vi "rsidr_core_global.vi"() -> ()   [LabVIEW 2020, in "Rohde&Schwarz RTx Oscilloscopes.lvlib"] (continued)
2"=0.0, "Command"="DESK"}]}, {"Type"=2, "Name"="rsrtx_rngScaleLinLog", "Entries"=[{"Name"="Linear", "Value 1"=0.0, "Value 2"=0.0, "Command"="LIN"}, {"Name"="Logarithmic", "Value 1"=1.0, "Value 2"=0.0, "Command"="LOG"}]}, {"Type"=2, "Name"="rsrtx_rngHarmonicsFundamentalMIL", "Entries"=[{"Name"="F60", "Value 1"=0.0, "Value 2"=0.0, "Command"="F60"}, {"Name"="F400", "Value 1"=1.0, "Value 2"=0.0, "Command"="F400"}]}, {"Type"=2, "Name"="rsrtx_rngHarmonicsFundamentalRTC", "Entries"=[{"Name"="F400", "Value 1"=0.0, "Value 2"=0.0, "Command"="F400"}, {"Name"="NVF", "Value 1"=1.0, "Value 2"=0.0, "Command"="NVF"}, {"Name"="WVF", "Value 1"=2.0, "Value 2"=0.0, "Command"="WVF"}]}, {"Type"=0, "Name"="rsrtx_rngPowerAnalysisReportTemperature", "Entries"=[{"Name"="", "Value 1"=-273.0, "Value 2"=32767.0, "Command"=""}]}, {"Type"=0, "Name"="rsrtx_rngTransientResponseSignal", "Entries"=[{"Name"="", "Value 1"=-10.0, "Value 2"=10.0, "Command"=""}]}, {"Type"=2, "Name"="rsrtx_rngProbeInputImpedance", "Entries"=[{"Name"="Unknown termination", "Value 1"=0.0, "Value 2"=0.0, "Command"="UNKN"}, {"Name"="50 Ohm termination", "Value 1"=1.0, "Value 2"=0.0, "Command"="50OH"}, {"Name"="1 M Ohm termination", "Value 1"=2.0, "Value 2"=0.0, "Command"="1MOH"}]}, {"Type"=2, "Name"="RsRtx_rngClockedSource", "Entries"=[{"Name"="D0", "Value 1"=0.0, "Value 2"=0.0, "Command"="D0"}, {"Name"="D1", "Value 1"=1.0, "Value 2"=0.0, "Command"="D1"}, {"Name"="D2", "Value 1"=2.0, "Value 2"=0.0, "Command"="D2"}, {"Name"="D3", "Value 1"=3.0, "Value 2"=0.0, "Command"="D3"}, {"Name"="D4", "Value 1"=4.0, "Value 2"=0.0, "Command"="D4"}, {"Name"="D5", "Value 1"=5.0, "Value 2"=0.0, "Command"="D5"}, {"Name"="D6", "Value 1"=6.0, "Value 2"=0.0, "Command"="D6"}, {"Name"="D7", "Value 1"=7.0, "Value 2"=0.0, "Command"="D7"}, {"Name"="D8", "Value 1"=8.0, "Value 2"=0.0, "Command"="D8"}, {"Name"="D9", "Value 1"=9.0, "Value 2"=0.0, "Command"="D9"}, {"Name"="D10", "Value 1"=10.0, "Value 2"=0.0, "Command"="D10"}, {"Name"="D11", "Value 1"=11.0, "Value 2"=0.0, "Command"="D11"}, {"Name"="D12", "Value 1"=12.0, "Value 2"=0.0, "Command"="D12"}, {"Name"="D13", "Value 1"=13.0, "Value 2"=0.0, "Command"="D13"}, {"Name"="D14", "Value 1"=14.0, "Value 2"=0.0, "Command"="D14"}, {"Name"="D15", "Value 1"=15.0, "Value 2"=0.0, "Command"="D15"}]}, {"Type"=2, "Name"="RsRtx_rngParallelBitSource", "Entries"=[{"Name"="D0", "Value 1"=0.0, "Value 2"=0.0, "Command"="D0"}, {"Name"="D1", "Value 1"=1.0, "Value 2"=0.0, "Command"="D1"}, {"Name"="D2", "Value 1"=2.0, "Value 2"=0.0, "Command"="D2"}, {"Name"="D3", "Value 1"=3.0, "Value 2"=0.0, "Command"="D3"}, {"Name"="D4", "Value 1"=4.0, "Value 2"=0.0, "Command"="D4"}, {"Name"="D5", "Value 1"=5.0, "Value 2"=0.0, "Command"="D5"}, {"Name"="D6", "Value 1"=6.0, "Value 2"=0.0, "Command"="D6"}, {"Name"="D7", "Value 1"=7.0, "Value 2"=0.0, "Command"="D7"}, {"Name"="D8", "Value 1"=8.0, "Value 2"=0.0, "Command"="D8"}, {"Name"="D9", "Value 1"=9.0, "Value 2"=0.0, "Command"="D9"}, {"Name"="D10", "Value 1"=10.0, "Value 2"=0.0, "Command"="D10"}, {"Name"="D11", "Value 1"=11.0, "Value 2"=0.0, "Command"="D11"}, {"Name"="D12", "Value 1"=12.0, "Value 2"=0.0, "Command"="D12"}, {"Name"="D13", "Value 1"=13.0, "Value 2"=0.0, "Command"="D13"}, {"Name"="D14", "Value 1"=14.0, "Value 2"=0.0, "Command"="D14"}, {"Name"="D15", "Value 1"=15.0, "Value 2"=0.0, "Command"="D15"}]}, {"Type"=0, "Name"="RsRtx_rngPctInt", "Entries"=[{"Name"="", "Value 1"=0.0, "Value 2"=100.0, "Command"=""}]}, {"Type"=2, "Name"="RsRtx_rngDVMType", "Entries"=[{"Name"="DC", "Value 1"=0.0, "Value 2"=0.0, "Command"="DC"}, {"Name"="AC DC RMS", "Value 1"=1.0, "Value 2"=0.0, "Command"="ACDC"}, {"Name"="AC RMS", "Value 1"=2.0, "Value 2"=0.0, "Command"="ACRM"}, {"Name"="Maximum", "Value 1"=3.0, "Value 2"=0.0, "Command"="UPE"}, {"Name"="Minimum", "Value 1"=4.0, "Value 2"=0.0, "Command"="LPE"}, {"Name"="Peak-to-Peak", "Value 1"=5.0, "Value 2"=0.0, "Command"="PEAK"}, {"Name"="Crest Factor", "Value 1"=6.0, "Value 2"=0.0, "Command"="CRES"}, {"Name"="Off", "Value 1"=7.0, "Value 2"=0.0, "Command"="OFF"}]}, {"Type"=2, "Name"="RsRtx_rngDVMPosition", "Entries"=[{"Name"="Top Left Corner", "Value 1"=0.0, "Value 2"=0.0, "Command"="TLEF"}, {"Name"="Top Right Corner", "Value 1"=1.0, "Value 2"=0.0, "Command"="TRIG"}, {"Name"="Bottom Left Corner", "Value 1"=2.0, "Value 2"=0.0, "Command"="BLEF"}, {"Name"="Bottom Right Corner", "Value 1"=3.0, "Value 2"=0.0, "Command"="BRIG"}]}, {"Type"=2, "Name"="RsRtx_rngMagnitudeScale", "Entries"=[{"Name"="Linear", "Value 1"=0.0, "Value 2"=0.0, "Command"="LIN"}, {"Name"="dBM", "Value 1"=1.0, "Value 2"=0.0, "Command"="DBM"}, {"Name"="dBV", "Value 1"=2.0, "Value 2"=0.0, "Command"="DBV"}, {"Name"="dBuV", "Value 1"=3.0, "Value 2"=0.0, "Command"="DBUV"}]}, {"Type"=2, "Name"="RsRtx_rngSpectrumFrequencyWindowType", "Entries"=[{"Name"="Rectangular", "Value 1"=0.0, "Value 2"=0.0, "Command"="RECT"}, {"Name"="Hamming", "Value 1"=1.0, "Value 2"=0.0, "Command"="HAMM"}, {"Name"="Hanning", "Value 1"=2.0, "Value 2"=0.0, "Command"="HANN"}, {"Name"="Blackman Harris", "Value 1"=3.0, "Value 2"=0.0, "Command"="BLAC"}, {"Name"="Flat Top", "Value 1"=4.0, "Value 2"=0.0, "Command"="FLAT"}]}, {"Type"=0, "Name"="RsRtx_rngSpectrumSpectrogramScale", "Entries"=[{"Name"="", "Value 1"=1.0, "Value 2"=20.0, "Command"=""}]}, {"Type"=2, "Name"="RsRtx_rngSpectrumMarkerDisplay", "Entries"=[{"Name"="Off", "Value 1"=0.0, "Value 2"=0.0, "Command"="OFF"}, {"Name"="Index", "Value 1"=1.0, "Value 2"=0.0, "Command"="IND"}, {"Name"="Result", "Value 1"=2.0, "Value 2"=0.0, "Command"="RES"}]}, {"Type"=2, "Name"="RsRtx_rngSpectrumMarkerSource", "Entries"=[{"Name"="Spectrum", "Value 1"=0.0, "Value 2"=0.0, "Command"="SPEC"}, {"Name"="Min Hold", "Value 1"=1.0, "Value 2"=0.0, "Command"="MINH"}, {"Name"="Max Hold", "Value 1"=2.0, "Value 2"=0.0, "Command"="MAXH"}, {"Name"="Average", "Value 1"=3.0, "Value 2"=0.0, "Command"="AVER"}]}, {"Type"=2, "Name"="RsRtx_rngSpectrumMarkerSetupDetectionMode", "Entries"=[{"Name"="Level Only", "Value 1"=0.0, "Value 2"=0.0, "Command"="LONL"}, {"Name"="Advanced", "Value 1"=1.0, "Value 2"=0.0, "Command"="ADV"}]}, {"Type"=2, "Name"="RsRtx_rngSpectrumMarkerReferenceMode", "Entries"=[{"Name"="Off", "Value 1"=0.0, "Value 2"=0.0, "Command"="OFF"}, {"Name"="Indicated", "Value 1"=1.0, "Value 2"=0.0, "Command"="IND"}, {"Name"="Range", "Value 1"=2.0, "Value 2"=0.0, "Command"="RANG"}]}, {"Type"=2, "Name"="RsRtx_rngSpectrumMarkerResultMode", "Entries"=[{"Name"="Absolute", "Value 1"=0.0, "Value 2"=0.0, "Command"="ABS"}, {"Name"="Frequency", "Value 1"=1.0, "Value 2"=0.0, "Command"="FREQ"}, {"Name"="Level", "Value 1"=2.0, "Value 2"=0.0, "Command"="LEV"}, {"Name"="Delta Level", "Value 1"=3.0, "Value 2"=0.0, "Command"="FLEV"}]}, {"Type"=2, "Name"="RsRtx_rngSpectrumMarkerTablePosition", "Entries"=[{"Name"="Top", "Value 1"=0.0, "Value 2"=0.0, "Command"="TOP"}, {"Name"="Bottom", "Value 1"=1.0, "Value 2"=0.0, "Command"="BOTT"}, {"Name"="Fullscreen", "Value 1"=2.0, "Value 2"=0.0, "Command"="FULL"}]}, {"Type"=2, "Name"="RsRtx_rngSpectrumDisplayColorScheme", "Entries"=[{"Name"="Monochrom", "Value 1"=0.0, "Value 2"=0.0, "Command"="MON"}, {"Name"="Temperature", "Value 1"=1.0, "Value 2"=0.0, "Command"="TEMP"}, {"Name"="Rainbow", "Value 1"=2.0, "Value 2"=0.0, "Command"="RAIN"}]}, {"Type"=2, "Name"="RsRtx_rngContentFormat", "Entries"=[{"Name"="All", "Value 1"=0.0, "Value 2"=0.0, "Command"="ALL"}, {"Name"="Without Attributes", "Value 1"=1.0, "Value 2"=0.0, "Command"="WTIM"}]}, {"Type"=2, "Name"="RsRtx_rngAcquisitionMode", "Entries"=[{"Name"="Refresh", "Value 1"=0.0, "Value 2"=0.0, "Command"="REFR"}, {"Name"="Average", "Value 1"=1.0, "Value 2"=0.0, "Command"="AVER"}, {"Name"="Envelope", "Value 1"=2.0, "Value 2"=0.0, "Command"="ENV"}]}, {"Type"=2, "Name"="RsRtx_rngAcquisitionState", "Entries"=[{"Name"="Run", "Value 1"=0.0, "Value 2"=0.0, "Command"="RUN"}, {"Name"="Stopping", "Value 1"=1.0, "Value 2"=0.0, "Command"="STOP"}, {"Name"="Complete", "Value 1"=2.0, "Value 2"=0.0, "Command"="COMP"}, {"Name"="Break", "Value 1"=3.0, "Value 2"=0.0, "Command"="BRE"}]}, {"Type"=2, "Name"="RsRtx_rngMathOperation", "Entries"=[{"Name"="Add", "Value 1"=0.0, "Value 2"=0.0, "Command"="ADD"}, {"Name"="Subtract", "Value 1"=1.0, "Value 2"=0.0, "Command"="SUB"}, {"Name"="Multiply", "Value 1"=2.0, "Value 2"=0.0, "Command"="MUL"}, {"Name"="Divide", "Value 1"=3.0, "Value 2"=0.0, "Command"="DIV"}]}, {"Type"=2, "Name"="rsrtx_rngMathSource", "Entries"=[{"Name"="Channel 1", "Value 1"=1.0, "Value 2"=0.0, "Command"="CH1"}, {"Name"="Channel 2", "Value 1"=2.0, "Value 2"=0.0, "Command"="CH2"}, {"Name"="Channel 3", "Value 1"=3.0, "Value 2"=0.0, "Command"="CH3"}, {"Name"="Channel 4", "Value 1"=4.0, "Value 2"=0.0, "Command"="CH4"}]}, {"Type"=2, "Name"="RsRtx_rngAbsoluteRelative", "Entries"=[{"Name"="Absolute", "Value 1"=0.0, "Value 2"=0.0, "Command"="ABS"}, {"Name"="Relative", "Value 1"=1.0, "Value 2"=0.0, "Command"="REL"}]}, {"Type"=2, "Name"="RsRtx_rngDeviceMode", "Entries"=[{"Name"="YT", "Value 1"=0.0, "Value 2"=0.0, "Command"="YT"}, {"Name"="Zoom", "Value 1"=1.0, "Value 2"=0.0, "Command"="ZOOM"}, {"Name"="XY", "Value 1"=2.0, "Value 2"=0.0, "Command"="XY"}, {"Name"="Quick Meas", "Value 1"=3.0, "Value 2"=0.0, "Command"="QME"}, {"Name"="Update", "Value 1"=4.0, "Value 2"=0.0, "Command"="UPD"}, {"Name"="Autoset", "Value 1"=5.0, "Value 2"=0.0, "Command"="AUT"}, {"Name"="MaskTest", "Value 1"=6.0, "Value 2"=0.0, "Command"="MASK"}, {"Name"="FFT", "Value 1"=7.0, "Value 2"=0.0, "Command"="FFT"}]}, {"Type"=2, "Name"="RsRtx_rngPersistenceType", "Entries"=[{"Name"="Off", "Value 1"=0.0, "Value 2"=0.0, "Command"="OFF"}, {"Name"="Time", "Value 1"=1.0, "Value 2"=0.0, "Command"="TIME"}, {"Name"="Infinite", "Value 1"=2.0, "Value 2"=0.0, "Command"="INF"}]}, {"Type"=2, "Name"="rsrtx_rngHardcopyFormat", "Entries"=[{"Name"="BMP", "Value 1"=1.0, "Value 2"=0.0, "Command"="BMP"}, {"Name"="PNG", "Value 1"=0.0, "Value 2"=0.0, "Command"="PNG"}, {"Name"="GIF", "Value 1"=2.0, "Value 2"=0.0, "Command"="GIF"}]}, {"Type"=0, "Name"="RsRtx_rngLogicCurrent", "Entries"=[{"Name"="", "Value 1"=0.0, "Value 2"=255.0, "Command"=""}]}, {"Type"=2, "Name"="RsRtx_rngLogicThreshold", "Entries"=[{"Name"="TTL", "Value 1"=0.0, "Value 2"=0.0, "Command"="TTL"}, {"Name"="ECL", "Value 1"=1.0, "Value 2"=0.0, "Command"="ECL"}, {"Name"="CMOS", "Value 1"=2.0, "Value 2"=0.0, "Command"="CMOS"}, {"Name"="User", "Value 1"=3.0, "Value 2"=0.0, "Command"="USER"}]}, {"Type"=2, "Name"="rsrtx_rngLogicHysteresis", "Entries"=[{"Name"="Small", "Value 1"=1.0, "Value 2"=0.0, "Command"="SMAL"}, {"Name"="Medium", "Value 1"=2.0, "Value 2"=0.0, "Command"="MED"}, {"Name"="Large", "Value 1"=3.0, "Value 2"=0.0, "Command"="LARG"}]}, {"Type"=2, "Name"="RsRtx_rngLogicType", "Entries"=[{"Name"="Sample", "Value 1"=0.0, "Value 2"=0.0, "Command"="SAMP"}, {"Name"="Peak Detect", "Value 1"=1.0, "Value 2"=0.0, "Command"="PDET"}]}, {"Type"=2, "Name"="RsRtx_rngWaveformGeneratorFunctionType", "Entries"=[{"Name"="Sinusoid", "Value 1"=0.0, "Value 2"=0.0, "Command"="SIN"}, {"Name"="Square", "Value 1"=1.0, "Value 2"=0.0, "Command"="SQU"}, {"Name"="Ramp", "Value 1"=2.0, "Value 2"=0.0, "Command"="RAMP"}, {"Name"="DC", "Value 1"=3.0, "Value 2"=0.0, "Command"="DC"}, {"Name"="Pulse", "Value 1"=4.0, "Value 2"=0.0, "Command"="PULS"}, {"Name"="Sinc", "Value 1"=5.0, "Value 2"=0.0, "Command"="SINC"}, {"Name"="Triangle", "Value 1"=6.0, "Value 2"=0.0, "Command"="TRI"}, {"Name"="Exponential", "Value 1"=7.0, "Value 2"=0.0, "Command"="EXP"}, {"Name"="Arbitrary", "Value 1"=8.0, "Value 2"=0.0, "Command"="ARB"}]}, {"Type"=0, "Name"="RsRtx_rngWaveformGeneratorDutyCycle", "Entries"=[{"Name"="", "Value 1"=10.0, "Value 2"=90.0, "Command"=""}]}, {"Type"=2, "Name"="RsRtx_rngWaveformGeneratorModulationType", "Entries"=[{"Name"="AM", "Value 1"=0.0, "Value 2"=0.0, "Command"="AM"}, {"Name"="FM", "Value 1"=1.0, "Value 2"=0.0, "Command"="FM"}, {"Name"="ASK", "Value 1"=2.0, "Value 2"=0.0, "Command"="ASK"}, {"Name"="FSK", "Value 1"=3.0, "Value 2"=0.0, "Command"="FSK"}]}, {"Type"=0, "Name"="RsRtx_rngPercent", "Entries"=[{"Name"="", "Value 1"=0.0, "Value 2"=100.0, "Command"=""}]}, {"Type"=2, "Name"="RsRtx_rngWaveformGeneratorArbitrarySource", "Entries"=[{"Name"="Channel 1", "Value 1"=1.0, "Value 2"=0.0, "Command"="CH1"}, {"Name"="Channel 2", "Value 1"=2.0, "Value 2"=0.0, "Command"="CH2"}, {"Name"="Channel 3", "Value 1"=3.0, "Value 2"=0.0, "Command"="CH3"}, {"Name"="Channel 4", "Value 1"=4.0, "Value 2"=0.0, "Command"="CH4"}]}, {"Type"=2, "Name"="RsRtx_rngWaveformGeneratorLoad", "Entries"=[{"Name"="Fifty Ohm", "Value 1"=0.0, "Value 2"=0.0, "Command"="R50"}, {"Name"="High-Z", "Value 1"=1.0, "Value 2"=0.0, "Command"="HIGH"}]}, {"Type"=2, "Name"="RsRtx_rngWaveformGeneratorModulationFunctionType", "Entries"=[{"Name"="Sinusoid", "Value 1"=0.0, "Value 2"=0.0, "Command"="SIN"}, {"Name"="Square", "Value 1"=1.0, "Value 2"=0.0, "Command"="SQU"}, {"Name"="Ramp", "Value 1"=2.0, "Value 2"=0.0, "Command"="RAMP"}, {"Name"="Triangle", "Value 1"=3.0, "Value 2"=0.0, "Command"="TRI"}]}, {"Type"=2, "Name"="RsRtx_rngWaveformGeneratorOutputDestination", "Entries"=[{"Name"="BNC", "Value 1"=0.0, "Value 2"=0.0, "Command"="BNC"}, {"Name"="P3", "Value 1"=1.0, "Value 2"=0.0, "Command"="P3"}]}, {"Type"=2, "Name"="RsRtx_rngPatternGeneratorFunctionType", "Entries"=[{"Name"="Square", "Value 1"=0.0, "Value 2"=0.0, "Command"="SQU"}, {"Name"="Counter", "Value 1"=1.0, "Value 2"=0.0, "Command"="COUN"}, {"Name"="Arbitrary", "Value 1"=2.0, "Value 2"=0.0, "Command"="ARB"}, {"Name"="SPI", "Value 1"=3.0, "Value 2"=0.0, "Command"="SPI"}, {"Name"="I2C", "Value 1"=4.0, "Value 2"=0.0, "Command"="I2C"}, {"Name"="UART", "Value 1"=5.0, "Value 2"=0.0, "Command"="UART"}, {"Name"="CAN", "Value 1"=6.0, "Value 2"=0.0, "Command"="CAN"}, {"Name"="LIN", "Value 1"=7.0, "Value 2"=0.0, "Command"="LIN"}, {"Name"="Manual", "Value 1"=8.0, "Value 2"=0.0, "Command"="MAN"}, {"Name"="Audio I2S", "Value 1"=9.0, "Value 2"=0.0, "Command"="I2S"}, {"Name"="Audio TDM", "Value 1"=10.0, "Value 2"=0.0, "Command"="TDM"}, {"Name"="Test Pulse Width", "Value 1"=11.0, "Value 2"=0.0, "Command"="TPWM"}, {"Name"="Pulse Width", "Value 1"=12.0, "Value 2"=0.0, "Command"="PWM"}, {"Name"="LED Pulse Width", "Value 1"=13.0, "Value 2"=0.0, "Command"="LEDP"}]}, {"Type"=2, "Name"="RsRtx_rngPatternGeneratorCounterDirection", "Entries"=[{"Name"="Downward", "Value 1"=0.0, "Value 2"=0.0, "Command"="DOWN"}, {"Name"="Upward", "Value 1"=1.0, "Value 2"=0.0, "Command"="UPW"}]}, {"Type"=2, "Name"="RsRtx_rngPatternGeneratorTriggerMode", "Entries"=[{"Name"="Continuous", "Value 1"=0.0, "Value 2"=0.0, "Command"="CONT"}, {"Name"="Single", "Value 1"=1.0, "Value 2"=0.0, "Command"="SING"}]}, {"Type"=2, "Name"="rsrtx_rngWindowRange", "Entries"=[{"Name"="Enter", "Value 1"=0.0, "Value 2"=0.0, "Command"="ENT"}, {"Name"="Exit", "Value 1"=1.0, "Value 2"=0.0, "Command"="EXI"}, {"Name"="Within", "Value 1"=2.0, "Value 2"=0.0, "Command"="WITH"}, {"Name"="Outside", "Value 1"=3.0, "Value 2"=0.0, "Command"="OUTS"}, {"Name"="Passthrough", "Value 1"=4.0, "Value 2"=0.0, "Command"="PASS"}, {"Name"="No Passthrough", "Value 1"=5.0, "Value 2"=0.0, "Command"="NPAS"}]}, {"Type"=2, "Name"="RsRtx_rngSpectrumAnalysisMode", "Entries"=[{"Name"="Spectrum", "Value 1"=0.0, "Value 2"=0.0, "Command"="SPEC"}, {"Name"="FFT", "Value 1"=1.0, "Value 2"=0.0, "Command"="FFT"}]}, {"Type"=2, "Name"="RsRtx_rngInterface", "Entries"=[{"Name"="Ethernet", "Value 1"=0.0, "Value 2"=0.0, "Command"="ETH"}, {"Name"="USB", "Value 1"=1.0, "Value 2"=0.0, "Command"="USB"}]}, {"Type"=2, "Name"="RsRtx_rngUSBClass", "Entries"=[{"Name"="TMC", "Value 1"=0.0, "Value 2"=0.0, "Command"="TMC"}, {"Name"="VCP", "Value 1"=1.0, "Value 2"=0.0, "Command"="VCP"}, {"Name"="MTP", "Value 1"=2.0, "Value 2"=0.0, "Command"="MTP"}]}, {"Type"=2, "Name"="RsRtx_rngEthernetTransfer", "Entries"=[{"Name"="Auto", "Value 1"=0.0, "Value 2"=0.0, "Command"="AUTO"}, {"Name"="FD10", "Value 1"=1.0, "Value 2"=0.0, "Command"="FD10"}, {"Name"="FD100", "Value 1"=2.0, "Value 2"=0.0, "Command"="FD100"}, {"Name"="HD10", "Value 1"=3.0, "Value 2"=0.0, "Command"="HD10"}, {"Name"="HD100", "Value 1"=4.0, "Value 2"=0.0, "Command"="HD100"}]}, {"Type"=2, "Name"="RsRtx_rngTimeoutRange", "Entries"=[{"Name"="Low", "Value 1"=0.0, "Value 2"=0.0, "Command"="LOW"}, {"Name"="High", "Value 1"=1.0, "Value 2"=0.0, "Command"="HIGH"}, {"Name"="Either", "Value 1"=2.0, "Value 2"=0.0, "Command"="EITH"}]}, {"Type"=0, "Name"="RsRtx_rngTimeoutTriggerTime", "Entries"=[{"Name"="", "Value 1"=6.4e-09, "Value 2"=13.7439, "Command"=""}]}, {"Type"=2, "Name"="RsRtx_rngMILSTDTriggerFrame", "Entries"=[{"Name"="Command", "Value 1"=0.0, "Value 2"=0.0, "Command"="COMM"}, {"Name"="Status", "Value 1"=1.0, "Value 2"=0.0, "Command"="STAT"}, {"Name"="Data", "Value 1"=2.0, "Value 2"=0.0, "Command"="DATA"}, {"Name"="All", "Value 1"=3.0, "Value 2"=0.0, "Command"="ALL"}]}, {"Type"=2, "Name"="RsRtx_rngPointSelection", "Entries"=[{"Name"="Default", "Value 1"=0.0, "Value 2"=0.0, "Command"="DEF"}, {"Name"="Maximum", "Value 1"=1.0, "Value 2"=0.0, "Command"="MAX"}, {"Name"="DisplayMaximum", "Value 1"=2.0, "Value 2"=0.0, "Command"="DMAX"}]}, {"Type"=2, "Name"="RsRtx_rngUARTTriggerSource", "Entries"=[{"Name"="RX", "Value 1"=0.0, "Value 2"=0.0, "Command"="RX"}, {"Name"="TX", "Value 1"=1.0, "Value 2"=0.0, "Command"="TX"}]}, {"Type"=2, "Name"="RsRtx_rngUARTFrameSource", "Entries"=[{"Name"="RX", "Value 1"=0.0, "Value 2"=0.0, "Command"="RX"}, {"Name"="TX", "Value 1"=1.0, "Value 2"=0.0, "Command"="TX"}]}, {"Type"=2, "Name"="rsrtx_rngSearchResultType", "Entries"=[{"Name"="Edge", "Value 1"=0.0, "Value 2"=0.0, "Command"="EDGE"}, {"Name"="Width", "Value 1"=1.0, "Value 2"=0.0, "Command"="WIDTH"}, {"Name"="Peak", "Value 1"=2.0, "Value 2"=0.0, "Command"="PEAK"}, {"Name"="Runt", "Value 1"=3.0, "Value 2"=0.0, "Command"="RUNT"}, {"Name"="Rise Time", "Value 1"=4.0, "Value 2"=0.0, "Command"="RTIM"}, {"Name"="Data2Clock", "Value 1"=5.0, "Value 2"=0.0, "Command"="DATATOCLOCK"}, {"Name"="Pattern", "Value 1"=6.0, "Value 2"=0.0, "Command"="PATTERN"}, {"Name"="Protocol", "Value 1"=7.0, "Value 2"=0.0, "Command"="PROTOCOL"}, {"Name"="Window", "Value 1"=8.0, "Value 2"=0.0, "Command"="WINDOW"}]}, {"Type"=2, "Name"="rsrtx_rngSearchResultSlope", "Entries"=[{"Name"="Rising Edge", "Value 1"=0.0, "Value 2"=0.0, "Command"="POSITIVE"}, {"Name"="Falling Edge", "Value 1"=1.0, "Value 2"=0.0, "Command"="NEGATIVE"}, {"Name"="Either", "Value 1"=2.0, "Value 2"=0.0, "Command"="EITHER"}]}, {"Type"=2, "Name"="RsRtx_rngMemoryMode", "Entries"=[{"Name"="Automatic", "Value 1"=0.0, "Value 2"=0.0, "Command"="AUT"}, {"Name"="Predefined", "Value 1"=1.0, "Value 2"=0.0, "Command"="DMEM"}, {"Name"="Manual", "Value 1"=2.0, "Value 2"=0.0, "Command"="MAN"}]}, {"Type"=2, "Name"="RsRtx_rngBodeAmplitudeMode", "Entries"=[{"Name"="Constant", "Value 1"=0.0, "Value 2"=0.0, "Command"="CONS"}, {"Name"="Profile", "Value 1"=1.0, "Value 2"=0.0, "Command"="PROF"}]}, {"Type"=0, "Name"="RsRtx_rngBodeAmplitudePosition", "Entries"=[{"Name"="", "Value 1"=-10.0, "Value 2"=10.0, "Command"=""}]}, {"Type"=0, "Name"="RsRtx_rngBodeAmplitudeProfilePoints", "Entries"=[{"Name"="", "Value 1"=2.0, "Value 2"=16.0, "Command"=""}]}, {"Type"=0, "Name"="RsRtx_rngBodeAmplitudeScale", "Entries"=[{"Name"="", "Value 1"=0.1, "Value 2"=2.0, "Command"=""}]}, {"Type"=0, "Name"="RsRtx_rngBodeGainPosition", "Entries"=[{"Name"="", "Value 1"=-20.0, "Value 2"=20.0, "Command"=""}]}, {"Type"=0, "Name"="RsRtx_rngBodeGainScale", "Entries"=[{"Name"="", "Value 1"=0.1, "Value 2"=20.0, "Command"=""}]}, {"Type"=0, "Name"="RsRtx_rngBodeMeasurementDelay", "Entries"=[{"Name"="", "Value 1"=0.0, "Value 2"=10.0, "Command"=""}]}, {"Type"=0, "Name"="RsRtx_rngBodePointsPerDecade", "Entries"=[{"Name"="", "Value 1"=10.0, "Value 2"=500.0, "Command"=""}]}, {"Type"=0, "Name"="RsRtx_rngChannelPosition", "Entries"=[{"Name"="", "Value 1"=-5.0, "Value 2"=5.0, "Command"=""}]}, {"Type"=0, "Name"="RsRtx_rngPWMDutyCycle", "Entries"=[{"Name"="", "Value 1"=1.0, "Value 2"=99.0, "Command"=""}]}, {"Type"=0, "Name"="RsRtx_rngProbeGain", "Entries"=[{"Name"="", "Value 1"=0.0001, "Value 2"=10000.0, "Command"=""}]}, {"Type"=0, "Name"="RsRtx_rng16BitRange", "Entries"=[{"Name"="", "Value 1"=0.0, "Value 2"=65535.0, "Command"=""}]}, {"Type"=0, "Name"="RsRtx_rngBurstIdleTime", "Entries"=[{"Name"="", "Value 1"=2.8e-08, "Value 2"=17.0, "Command"=""}]}, {"Type"=0, "Name"="RsRtx_rngBurstCycles", "Entries"=[{"Name"="", "Value 1"=1.0, "Value 2"=1023.0, "Command"=""}]}, {"Type"=0, "Name"="RsRtx_rng360Degrees", "Entries"=[{"Name"="", "Value 1"=0.0, "Value 2"=360.0, "Command"=""}]}, {"Type"=0, "Name"="RsRtx_rngTriangleSymmetry", "Entries"=[{"Name"="", "Value 1"=1.0, "Value 2"=99.0, "Command"=""}]}, {"Type"=0, "Name"="RsRtx_rngBodePlotStartFrequency", "Entries"=[{"Name"="", "Value 1"=10.0, "Value 2"=25000000.0, "Command"=""}]}, {"Type"=0, "Name"="RsRtx_rngBodePlotStopFrequency", "Entries"=[{"Name"="", "Value 1"=10.0, "Value 2"=25000000.0, "Command"=""}]}, {"Type"=2, "Name"="RsRtx_rngBodeSourceChannel", "Entries"=[{"Name"="Channel 1", "Value 1"=0.0, "Value 2"=0.0, "Command"="CH1"}, {"Name"="Channel 2", "Value 1"=1.0, "Value 2"=0.0, "Command"="CH2"}, {"Name"="Channel 3", "Value 1"=2.0, "Value 2"=0.0, "Command"="CH3"}, {"Name"="Channel 4", "Value 1"=3.0, "Value 2"=0.0, "Command"="CH4"}]}, {"Type"=2, "Name"="RsRtx_rngBodePlotMeasurementState", "Entries"=[{"Name"="Stop", "Value 1"=0.0, "Value 2"=0.0, "Command"="STOP"}, {"Name"="Run", "Value 1"=1.0, "Value 2"=0.0, "Command"="RUN"}]}, {"Type"=0, "Name"="RsRtx_rngBodePhasePosition", "Entries"=[{"Name"="", "Value 1"=-20.0, "Value 2"=20.0, "Command"=""}]}, {"Type"=0, "Name"="RsRtx_rngBodePhaseScale", "Entries"=[{"Name"="", "Value 1"=0.1, "Value 2"=45.0, "Command"=""}]}, {"Type"=2, "Name"="RsRtx_rngUARTFrameState", "Entries"=[{"Name"="OK", "Value 1"=0.0, "Value 2"=0.0, "Command"="OK"}, {"Name"="Start Error", "Value 1"=1.0, "Value 2"=0.0, "Command"="STER"}, {"Name"="Stop Error", "Value 1"=2.0, "Value 2"=0.0, "Command"="SPER"}, {"Name"="Parity Error", "Value 1"=3.0, "Value 2"=0.0, "Command"="PRER"}, {"Name"="Break Condition", "Value 1"=4.0, "Value 2"=0.0, "Command"="BRE"}, {"Name"="Incomplete", "Value 1"=5.0, "Value 2"=0.0, "Command"="INS"}]}, {"Type"=2, "Name"="RsRtx_rngIdleStatePolarity", "Entries"=[{"Name"="Idle High", "Value 1"=0.0, "Value 2"=0.0, "Command"="IDLH"}, {"Name"="Idle Low", "Value 1"=1.0, "Value 2"=0.0, "Command"="IDLL"}]}, {"Type"=2, "Name"="RsRtx_rngMathWaveformColor", "Entries"=[{"Name"="Default", "Value 1"=0.0, "Value 2"=0.0, "Command"="DEF"}, {"Name"="Temperature", "Value 1"=1.0, "Value 2"=0.0, "Command"="TEMP"}, {"Name"="Rainbow", "Value 1"=2.0, "Value 2"=0.0, "Command"="RAIN"}, {"Name"="Fire", "Value 1"=3.0, "Value 2"=0.0, "Command"="FIRE"}, {"Name"="Yellow", "Value 1"=4.0, "Value 2"=0.0, "Command"="YELL"}, {"Name"="Green", "Value 1"=5.0, "Value 2"=0.0, "Command"="GRE"}, {"Name"="Orange", "Value 1"=6.0, "Value 2"=0.0, "Command"="ORAN"}, {"Name"="Blue", "Value 1"=7.0, "Value 2"=0.0, "Command"="BLUE"}, {"Name"="Light blue", "Value 1"=8.0, "Value 2"=0.0, "Command"="LBL"}, {"Name"="White", "Value 1"=9.0, "Value 2"=0.0, "Command"="WHIT"}, {"Name"="Cyan", "Value 1"=10.0, "Value 2"=0.0, "Command"="CYAN"}, {"Name"="Pink", "Value 1"=11.0, "Value 2"=0.0, "Command"="PINK"}, {"Name"="Red", "Value 1"=12.0, "Value 2"=0.0, "Command"="RED"}]}, {"Type"=2, "Name"="RsRtx_rngChannelWaveformColor", "Entries"=[{"Name"="Default", "Value 1"=0.0, "Value 2"=0.0, "Command"="DEF"}, {"Name"="Temperature", "Value 1"=1.0, "Value 2"=0.0, "Command"="TEMP"}, {"Name"="Rainbow", "Value 1"=2.0, "Value 2"=0.0, "Command"="RAIN"}, {"Name"="Fire", "Value 1"=3.0, "Value 2"=0.0, "Command"="FIRE"}]}, {"Type"=2, "Name"="RsRtx_rngMaskCaptureMode", "Entries"=[{"Name"="All", "Value 1"=0.0, "Value 2"=0.0, "Command"="ALL"}, {"Name"="Failed", "Value 1"=1.0, "Value 2"=0.0, "Command"="FAIL"}]}, {"Type"=2, "Name"="RsRtx_rngPWMMotorDirection", "Entries"=[{"Name"="Positive", "Value 1"=0.0, "Value 2"=0.0, "Command"="POS"}, {"Name"="Negative", "Value 1"=1.0, "Value 2"=0.0, "Command"="NEG"}]}, {"Type"=2, "Name"="RsRtx_rngReferenceWaveformColor", "Entries"=[{"Name"="Default", "Value 1"=0.0, "Value 2"=0.0, "Command"="DEF"}, {"Name"="Temperature", "Value 1"=1.0, "Value 2"=0.0, "Command"="TEMP"}, {"Name"="Rainbow", "Value 1"=2.0, "Value 2"=0.0, "Command"="RAIN"}, {"Name"="Fire", "Value 1"=3.0, "Value 2"=0.0, "Command"="FIRE"}, {"Name"="Yellow", "Value 1"=4.0, "Value 2"=0.0, "Command"="YELL"}, {"Name"="Green", "Value 1"=5.0, "Value 2"=0.0, "Command"="GRE"}, {"Name"="Orange", "Value 1"=6.0, "Value 2"=0.0, "Command"="ORAN"}, {"Name"="Blue", "Value 1"=7.0, "Value 2"=0.0, "Command"="BLUE"}, {"Name"="Light blue", "Value 1"=8.0, "Value 2"=0.0, "Command"="LBL"}, {"Name"="White", "Value 1"=9.0, "Value 2"=0.0, "Command"="WHIT"}, {"Name"="Cyan", "Value 1"=10.0, "Value 2"=0.0, "Command"="CYAN"}, {"Name"="Pink", "Value 1"=11.0, "Value 2"=0.0, "Command"="PINK"}, {"Name"="Red", "Value 1"=12.0, "Value 2"=0.0, "Command"="RED"}]}, {"Type"=0, "Name"="RsRtx_rngEthernetIPPort", "Entries"=[{"Name"="", "Value 1"=1024.0, "Value 2"=65535.0, "Command"=""}]}, {"Type"=2, "Name"="RsRtx_rngCounterSource", "Entries"=[{"Name"="Trigger", "Value 1"=0.0, "Value 2"=0.0, "Command"="TRIG"}, {"Name"="Channel 1", "Value 1"=1.0, "Value 2"=0.0, "Command"="CH1"}, {"Name"="Channel 2", "Value 1"=2.0, "Value 2"=0.0, "Command"="CH2"}, {"Name"="Channel 3", "Value 1"=3.0, "Value 2"=0.0, "Command"="CH3"}, {"Name"="Channel 4", "Value 1"=4.0, "Value 2"=0.0, "Command"="CH4"}]}, {"Type"=0, "Name"="rsrtx_rngProtocolLINDataLength", "Entries"=[{"Name"="", "Value 1"=1.0, "Value 2"=8.0, "Command"=""}]}, {"Type"=2, "Name"="rsrtx_rngWaveformExportParameter", "Entries"=[{"Name"="Channel 1", "Value 1"=1.0, "Value 2"=0.0, "Command"="CH1"}, {"Name"="Channel 2", "Value 1"=2.0, "Value 2"=0.0, "Command"="CH2"}, {"Name"="Channel 3", "Value 1"=3.0, "Value 2"=0.0, "Command"="CH3"}, {"Name"="Channel 4", "Value 1"=4.0, "Value 2"=0.0, "Command"="CH4"}, {"Name"="Math Waveform 1", "Value 1"=5.0, "Value 2"=0.0, "Command"="MA1"}, {"Name"="Math Waveform 2", "Value 1"=6.0, "Value 2"=0.0, "Command"="MA2"}, {"Name"="Math Waveform 3", "Value 1"=7.0, "Value 2"=0.0, "Command"="MA3"}, {"Name"="Math Waveform 4", "Value 1"=8.0, "Value 2"=0.0, "Command"="MA4"}, {"Name"="Math Waveform 5", "Value 1"=9.0, "Value 2"=0.0, "Command"="MA5"}, {"Name"="Reference Waveform 1", "Value 1"=10.0, "Value 2"=0.0, "Command"="RE1"}, {"Name"="Reference Waveform 2", "Value 1"=11.0, "Value 2"=0.0, "Command"="RE2"}, {"Name"="Reference Waveform 3", "Value 1"=12.0, "Value 2"=0.0, "Command"="RE3"}, {"Name"="Reference Waveform 4", "Value 1"=13.0, "Value 2"=0.0, "Command"="RE4"}, {"Name"="Digital 70", "Value 1"=30.0, "Value 2"=0.0, "Command"="D70"}, {"Name"="Digital 158", "Value 1"=31.0, "Value 2"=0.0, "Command"="D158"}]}, {"Type"=2, "Name"="rsrtx_rngReferenceWaveformParameter", "Entries"=[{"Name"="Channel 1", "Value 1"=1.0, "Value 2"=0.0, "Command"="CH1"}, {"Name"="Channel 2", "Value 1"=2.0, "Value 2"=0.0, "Command"="CH2"}, {"Name"="Channel 3", "Value 1"=3.0, "Value 2"=0.0, "Command"="CH3"}, {"Name"="Channel 4", "Value 1"=4.0, "Value 2"=0.0, "Command"="CH4"}, {"Name"="Math Waveform 1", "Value 1"=5.0, "Value 2"=0.0, "Command"="MA1"}, {"Name"="Math Waveform 2", "Value 1"=6.0, "Value 2"=0.0, "Command"="MA2"}, {"Name"="Math Waveform 3", "Value 1"=7.0, "Value 2"=0.0, "Command"="MA3"}, {"Name"="Math Waveform 4", "Value 1"=8.0, "Value 2"=0.0, "Command"="MA4"}, {"Name"="Math Waveform 5", "Value 1"=9.0, "Value 2"=0.0, "Command"="MA5"}, {"Name"="Reference Waveform 1", "Value 1"=10.0, "Value 2"=0.0, "Command"="RE1"}, {"Name"="Reference Waveform 2", "Value 1"=11.0, "Value 2"=0.0, "Command"="RE2"}, {"Name"="Reference Waveform 3", "Value 1"=12.0, "Value 2"=0.0, "Command"="RE3"}, {"Name"="Reference Waveform 4", "Value 1"=13.0, "Value 2"=0.0, "Command"="RE4"}, {"Name"="Digital 70", "Value 1"=30.0, "Value 2"=0.0, "Command"="D70"}, {"Name"="Digital 158", "Value 1"=31.0, "Value 2"=0.0, "Command"="D158"}, {"Name"="Spectrum", "Value 1"=32.0, "Value 2"=0.0, "Command"="SPEC"}, {"Name"="Minimum Hold", "Value 1"=34.0, "Value 2"=0.0, "Command"="MINH"}, {"Name"="Maximum Hold", "Value 1"=35.0, "Value 2"=0.0, "Command"="MAXH"}, {"Name"="Average", "Value 1"=36.0, "Value 2"=0.0, "Command"="AVER"}]}, {"Type"=0, "Name"="RsRtx_rngProbeZeroAdjust", "Entries"=[{"Name"="", "Value 1"=-100.0, "Value 2"=100.0, "Command"=""}]}, {"Type"=2, "Name"="RsRtx_rngProbeInputVoltageRange", "Entries"=[{"Name"="Auto", "Value 1"=0.0, "Value 2"=0.0, "Command"="AUTO"}, {"Name"="High", "Value 1"=1.0, "Value 2"=0.0, "Command"="MHIG"}, {"Name"="Low", "Value 1"=2.0, "Value 2"=0.0, "Command"="MLOW"}]}, {"Type"=2, "Name"="RsRtx_rngProbeMeasMode", "Entries"=[{"Name"="Differential", "Value 1"=0.0, "Value 2"=0.0, "Command"="DMOD"}, {"Name"="Common", "Value 1"=1.0, "Value 2"=0.0, "Command"="CMOD"}, {"Name"="Positive", "Value 1"=2.0, "Value 2"=0.0, "Command"="PMOD"}, {"Name"="Negative", "Value 1"=3.0, "Value 2"=0.0, "Command"="NMOD"}]}, {"Type"=2, "Name"="RsRtx_rngMeasurementDelayDirection", "Entries"=[{"Name"="Nearest", "Value 1"=0.0, "Value 2"=0.0, "Command"="NEAR"}, {"Name"="Forward", "Value 1"=1.0, "Value 2"=0.0, "Command"="FRFI"}, {"Name"="Backward", "Value 1"=2.0, "Value 2"=0.0, "Command"="FRLA"}]}, {"Type"=2, "Name"="RsRtx_rngBurstTriggerMode", "Entries"=[{"Name"="Continuous", "Value 1"=0.0, "Value 2"=0.0, "Command"="CONT"}, {"Name"="Single", "Value 1"=1.0, "Value 2"=0.0, "Command"="SING"}]}, {"Type"=2, "Name"="RsRtx_rngChannelAndDigitalSource", "Entries"=[{"Name"="Channel 1", "Value 1"=1.0, "Value 2"=0.0, "Command"="CH1"}, {"Name"="Channel 2", "Value 1"=2.0, "Value 2"=0.0, "Command"="CH2"}, {"Name"="Channel 3", "Value 1"=3.0, "Value 2"=0.0, "Command"="CH3"}, {"Name"="Channel 4", "Value 1"=4.0, "Value 2"=0.0, "Command"="CH4"}, {"Name"="Digital Channel 0", "Value 1"=5.0, "Value 2"=0.0, "Command"="D0"}, {"Name"="Digital Channel 1", "Value 1"=6.0, "Value 2"=0.0, "Command"="D1"}, {"Name"="Digital Channel 2", "Value 1"=7.0, "Value 2"=0.0, "Command"="D2"}, {"Name"="Digital Channel 3", "Value 1"=8.0, "Value 2"=0.0, "Command"="D3"}, {"Name"="Digital Channel 4", "Value 1"=9.0, "Value 2"=0.0, "Command"="D4"}, {"Name"="Digital Channel 5", "Value 1"=10.0, "Value 2"=0.0, "Command"="D5"}, {"Name"="Digital Channel 6", "Value 1"=11.0, "Value 2"=0.0, "Command"="D6"}, {"Name"="Digital Channel 7", "Value 1"=12.0, "Value 2"=0.0, "Command"="D7"}, {"Name"="Digital Channel 8", "Value 1"=13.0, "Value 2"=0.0, "Command"="D8"}, {"Name"="Digital Channel 9", "Value 1"=14.0, "Value 2"=0.0, "Command"="D9"}, {"Name"="Digital Channel 10", "Value 1"=15.0, "Value 2"=0.0, "Command"="D10"}, {"Name"="Digital Channel 11", "Value 1"=16.0, "Value 2"=0.0, "Command"="D11"}, {"Name"="Digital Channel 12", "Value 1"=17.0, "Value 2"=0.0, "Command"="D12"}, {"Name"="Digital Channel 13", "Value 1"=18.0, "Value 2"=0.0, "Command"="D13"}, {"Name"="Digital Channel 14", "Value 1"=19.0, "Value 2"=0.0, "Command"="D14"}, {"Name"="Digital Channel 15", "Value 1"=20.0, "Value 2"=0.0, "Command"="D15"}]}, {"Type"=2, "Name"="rsrtx_rngWaveformGeneratorSweepType", "Entries"=[{"Name"="Linear", "Value 1"=0.0, "Value 2"=0.0, "Command"="LIN"}, {"Name"="Logarithmic", "Value 1"=1.0, "Value 2"=0.0, "Command"="LOG"}, {"Name"="Triangle", "Value 1"=2.0, "Value 2"=0.0, "Command"="TRI"}]}] {"Type" items=["Range", "Coerced", "Discrete"]}
  in  "Attributes":T3[](array[typedef])=[{"Level"=1, "Class Only"=TRUE, "Identifier"="", "Descriptive Name"="Acquisition", "Data Type"=0, "Command"="", "Access"=0, "Range Table"="", "Read Callback"="", "Write Callback"="", "Supported Models"="", "Instrument Options"="", "Flags"=0, "Help"="This class contains attributes that configure the acquisition subsystem."}, {"Level"=2, "Class Only"=FALSE, "Identifier"="RSRTX_ATTR_RECORD_LENGTH_AUTOMATIC", "Descriptive Name"="Record Length Automatic", "Data Type"=3, "Command"="ACQ:POIN:AUT", "Access"=2, "Range Table"="", "Read Callback"="", "Write Callback"="", "Supported Models"="", "Instrument Options"="", "Flags"=0, "Help"="Enables or disables the automatic record length. The instrument sets a value that fits to the selected timebase.\n\nAvailable Repeated Capabilities:\nNone\n\nRemote-control command(s):\nACQuire:POINts:AUTomatic"}, {"Level"=2, "Class Only"=FALSE, "Identifier"="RSRTX_ATTR_RECORD_LENGTH", "Descriptive Name"="Record Length", "Data Type"=0, "Command"="ACQ:POIN", "Access"=2, "Range Table"="", "Read Callback"="", "Write Callback"="", "Supported Models"="", "Instrument Options"="", "Flags"=0, "Help"="Defines a record length value, the number of recorded waveform points in a segment.\n\nAvailable Repeated Capabilities:\nNone\n\nRemote-control command(s):\nACQuire:POINts[:VALue]"}, {"Level"=2, "Class Only"=FALSE, "Identifier"="RSRTX_ATTR_ACQUIRE_MODE", "Descriptive Name"="Acquire Mode", "Data Type"=0, "Command"="ACQ:TYPE", "Access"=2, "Range Table"="RsRtx_rngAcquisitionMode", "Read Callback"="", "Write Callback"="", "Supported Models"="RTB", "Instrument Options"="", "Flags"=0, "Help"="Sets the type of the aquisition mode.\n\nAvailable Repeated Capabilities:\nNone\n\nRemote-control command(s):\nACQuire:TYPE"}, {"Level"=2, "Class Only"=FALSE, "Identifier"="RSRTX_ATTR_PEAK_DETECT", "Descriptive Name"="Peak Detect", "Data Type"=3, "Command"="ACQ:PEAK", "Access"=2, "Range Table"="", "Read Callback"="rsrtx_OffOrAutoBool_ReadCallback.vi", "Write Callback"="rsrtx_OffOrAutoBool_WriteCallback.vi", "Supported Models"="", "Instrument Options"="", "Flags"=0, "Help"="Enables or disables the peak detect acquisition mode.\n\nAvailable Repeated Capabilities:\nNone\n\nRemote-control command(s):\nACQuire:PEAKdetect"}, {"Level"=2, "Class Only"=FALSE, "Identifier"="RSRTX_ATTR_HIGH_RESOLUTION", "Descriptive Name"="High Resolution", "Data Type"=3, "Command"="ACQ:HRES", "Access"=2, "Range Table"="", "Read Callback"="rsrtx_OffOrAutoBool_ReadCallback.vi", "Write Callback"="rsrtx_OffOrAutoBool_WriteCallback.vi", "Supported Models"="", "Instrument Options"="", "Flags"=0, "Help"="Enables or disables the high resolution acquisition mode.\n\nAvailable Repeated Capabilities:\nNone\n\nRemote-control command(s):\nACQuire:HRESolution"}, {"Level"=2, "Class Only"=FALSE, "Identifier"="RSRTX_ATTR_INTERPOLATION", "Descriptive Name"="Interpolation", "Data Type"=0, "Command"="ACQ:INT", "Access"=2, "Range Table"="rsrtx_rngInterpolation", "Read Callback"="", "Write Callback"="", "Supported Models"="", "Instrument Options"="", "Flags"=0, "Help"="Selects the interpolation method if ACQuire:MODE ITIMe (interpolated time) is set for enhancement.\n\nAvailable Repeated Capabilities:\nNone\n\nRemote-control command(s):\nACQuire:INTerpolate"}, {"Level"=2, "Class Only"=FALSE, "Identifier"="RSRTX_ATTR_NUM_AVERAGES", "Descriptive Name"="Number of Averages", "Data Type"=0, "Command"="ACQ:AVER:COUN", "Access"=2, "Range Table"="rsrtx_rngNumberofAverages", "Read Callback"="", "Write Callback"="", "Supported Models"="", "Instrument Options"="", "Flags"=0, "Help"="Defines the Average count that has a double effect:\n- it defines the number of waveforms used to calculate the average waveform, and\n- it sets the number of waveforms acquired with RUNSingle.\n\nAvailable Repeated Capabilities:\nNone\n\nRemote-control command(s):\nACQuire:AVERage:COUNt"}, {"Level"=2, "Class Only"=FALSE, "Identifier"="RSRTX_ATTR_NUM_AVERAGES_CURRENT", "Descriptive Name"="Number of Averages Current", "Data Type"=0, "Command"="ACQ:AVER:CURR?", "Access"=0, "Range Table"="", "Read Callback"="", "Write Callback"="", "Supported Models"="", "Instrument Options"="", "Flags"=0, "Help"="Returns the current amount of acquired waveforms that contribute to the average. The value is independent of the number of available segments, there are more waveforms in the average available than segments in history. Minimum is 2; maximum depends on the instrument settings.\n\nAvailable Repeated Capabilities:\nNone\n\nRemote-control command(s):\nACQuire:AVERage:CURRent?"}, {"Level"=2, "Class Only"=FALSE, "Identifier"="RSRTX_ATTR_NUM_AVERAGES_RESET", "Descriptive Name"="Number of Averages Reset", "Data Type"=4, "Command"="ACQ:AVER:RES", "Access"=1, "Range Table"="", "Read Callback"="", "Write Callback"="", "Supported Models"="", "Instrument Options"="", "Flags"=0, "Help"="Deletes the waveform and restarts the average calculation.\n\nAvailable Repeated Capabilities:\nNone\n\nRemote-control command(s):\nACQuire:AVERage:RESet"}, {"Level"=2, "Class Only"=FALSE, "Identifier"="RSRTX_ATTR_MEMORY_MODE", "Descriptive Name"="Memory Mode", "Data Type"=0, "Command"="ACQ:MEM", "Access"=2, "Range Table"="RsRtx_rngMemoryMode", "Read Callback"="", "Write Callback"="", "Supported Models"="", "Instrument Options"="", "Flags"=0, "Help"="Defines how the record length is set.\n\nAvailable Repeated Capabilities:\nNone\n\nRemote-control command(s):\nACQuire:MEMory[:MODE]"}, {"Level"=2, "Class Only"=FALSE, "Identifier"="RSRTX_ATTR_AVERAGING_STATUS", "Descriptive Name"="Averaging Status", "Data Type"=3, "Command"="ACQ:AVER:COMP?", "Access"=0, "Range Table"="", "Read Callback"="", "Write Callback"="", "Supported Models"="", "Instrument Options"="", "Flags"=0, "Help"="Returns the state of averaging.\nFalse - The number of acquired waveforms is less than the number required for average calculation. See RSRTX_ATTR_NUM_AVERAGES.\nTrue - The instrument acquired a sufficient number of waveforms to determine the average.\n\nAvailable Repeated Capabilities:\nNone\n\nRemote-control command(s):\nACQuire:AVERage:COMPlete?"}, {"Level"=2, "Class Only"=FALSE, "Identifier"="RSRTX_ATTR_NUMBER_OF_WAVEFORMS", "Descriptive Name"="Number Of Waveforms", "Data Type"=0, "Command"="ACQ:NSIN:COUN", "Access"=2, "Range Table"="rsrtx_rngNumberOfWaveforms", "Read Callback"="", "Write Callback"="", "Supported Models"="", "Instrument Options"="", "Flags"=0, "Help"="Sets the number of waveforms acquired with RUNSingle .\n\nAvailable Repeated Capabilities:\nNone\n\nRemote-control command(s):\nACQuire:NSINgle:COUNt"}, {"Level"=2, "Class Only"=FALSE, "Identifier"="RSRTX_ATTR_SAMPLE_MODE", "Descriptive Name"="Sample Mode", "Data Type"=0, "Command"="ACQ:MODE", "Access"=2, "Range Table"="rsrtx_rngSampleMode", "Read Callback"="", "Write Callback"="", "Supported Models"="", "Instrument Options"="", "Flags"=0, "Help"="Selects the method of adding waveform points to the samples of the ADC in order to fill the record length.\n\nAvailable Repeated Capabilities:\nNone\n\nRemote-control command(s):\nACQuire:MODE"}, {"Level"=2, "Class Only"=FALSE, "Identifier"="RSRTX_ATTR_WAVEFORM_RATE_MAXIMUM", "Descriptive Name"="Waveform Rate Maximum", "Data Type"=3, "Command"="ACQ:WRAT:MAX", "Access"=2, "Range Table"="", "Read Callback"="", "Write Callback"="", "Supported Models"="", "Instrument Options"="", "Flags"=0, "Help"="Enables/disables maximum waveform rate.\n\nAvailable Repeated Capabilities:\nNone\n\nRemote-control command(s):\nACQuire:WRATe:MAXimum"}, {"Level"=2, "Class Only"=FALSE, "Identifier"="RSRTX_ATTR_HORZ_TIME_PER_RECORD", "Descriptive Name"="Horizontal Time Per Record", "Data Type"=1, "Command"="TIM:ACQT", "Access"=2, "Range Table"="rsrtx_rngHorzAcquisitionTime", "Read Callback"="", "Write Callback"="", "Supported Models"="", "Instrument Options"="", "Flags"=0, "Help"="Defines the time of one acquisition, that is the time across the 10 divisions of the diagram: Horizontal Scale *10.\n\nAvailable Repeated Capabilities:\nNone\n\nRemote-control command(s):\nTIMebase:ACQTime"}, {"Level"=2, "Class Only"=FALSE, "Identifier"="RSRTX_ATTR_HORZ_SCALE", "Descriptive Name"="Horizontal Scale", "Data Type"=1, "Command"="TIM:SCAL", "Access"=2, "Range Table"="rsrtx_rngHorzScale", "Read Callback"="", "Write Callback"="", "Supported Models"="", "Instrument Options"="", "Flags"=0, "Help"="Sets the horizontal scale - the time per division on the x-axis - for all channel and math waveforms.\nThe setting accuracy depends on the current resolution (sample rate) and the setting for resolution enhancement:\n- In interpolated time mode if sample rate > ADC sample rate: Any value for the horizontal scale can be set due to the interpolation factor.\n- In real time mode and equivalent time mode for all sample rates; and in interpolated time mode if sample rate < ADC sample rate: The resolution is an integer multiple of the ADC sample rate.\n\nAvailable Repeated Capabilities:\nNone\n\nRemote-control command(s):\nTIMebase:SCALe"}, {"Level"=2, "Class Only"=FALSE, "Identifier"="RSRTX_ATTR_ROLL_MODE_AUTOMATIC", "Descriptive Name"="Roll Mode Automatic", "Data Type"=3, "Command"="TIM:ROLL:AUT", "Access"=2, "Range Table"="", "Read Callback"="", "Write Callback"="", "Supported Models"="", "Instrument Options"="", "Flags"=0, "Help"="Enables the automatic roll mode. The instrument switches to roll mode if the timebase is equal or slower than the roll mode limit defined with RSRTX_ATTR_ROLL_MODE_MINIMUM_TIME_BASE.\n\nAvailable Repeated Capabilities:\nNone\n\nRemote-control command(s):\nTIMebase:ROLL:AUTomatic"}, {"Level"=2, "Class Only"=FALSE, "Identifier"="RSRTX_ATTR_ROLL_MODE_MINIMUM_TIME_BASE", "Descriptive Name"="Roll Mode Minimum Time Base", "Data Type"=1, "Command"="TIM:ROLL:MTIM", "Access"=2, "Range Table"="", "Read Callback"="", "Write Callback"="", "Supported Models"="", "Instrument Options"="", "Flags"=0, "Help"="The roll mode is enabled automatically if the time base exceeds the MinTimeBase, and if RSRTX_ATTR_ROLL_MODE_AUTOMATIC is set ON.\n\nAvailable Repeated Capabilities:\nNone\n\nRemote-control command(s):\nTIMebase:ROLL:MTIMe"}, {"Level"=2, "Class Only"=FALSE, "Identifier"="RSRTX_ATTR_ACQUSITION_START_TIME", "Descriptive Name"="Acqusition Start Time", "Data Type"=1, "Command"="TIM:POS", "Access"=2, "Range Table"="rsrtx_rngAcquisitionStartTime", "Read Callback"="", "Write Callback"="", "Supported Models"="", "Instrument Options"="", "Flags"=0, "Help"="Defines the trigger offset - the time interval between trigger point and reference point to analyze the signal some time before or after the trigger event.\n\nAvailable Repeated Capabilities:\nNone\n\nRemote-control command(s):\nTIMebase:POSition"}, {"Level"=2, "Class Only"=FALSE, "Identifier"="RSRTX_ATTR_ACQUISITION_TIME", "Descriptive Name"="Acquisition Time", "Data Type"=1, "Command"="TIM:RAT?", "Access"=0, "Range Table"="", "Read Callback"="", "Write Callback"="", "Supported Models"="", "Instrument Options"="", "Flags"=0, "Help"="Queries the required acquisition time. If FFT gating is used and the resolution BW is set to constant, record length can be extended to acquire the required number of samples. In this case, the required acquisition time differs from the adjusted acquisition time.\n\nAvailable Repeated Capabilities:\nNone\n\nRemote-control command(s):\nTIMebase:RATime?"}, {"Level"=2, "Class Only"=FALSE, "Identifier"="RSRTX_ATTR_HORZ_ADC_SAMPLE_RATE", "Descriptive Name"="Horizontal ADC Sample Rate", "Data Type"=1, "Command"="ACQ:POIN:ARAT?", "Access"=0, "Range Table"="", "Read Callback"="", "Write Callback"="", "Supported Models"="", "Instrument Options"="", "Flags"=0, "Help"="Retrieves the sample rate of the ADC, that is the number of points that are sampled by the ADC in one second.\n\nAvailable Repeated Capabilities:\nNone\n\nRemote-control command(s):\nACQuire:POINts:ARATe?"}, {"Level"=2, "Class Only"=FALSE, "Identifier"="RSRTX_ATTR_HORZ_SAMPLE_RATE", "Descriptive Name"="Sample Rate", "Data Type"=1, "Command"="ACQ:SRAT?", "Access"=0, "Range Table"="", "Read Callback"="", "Write Callback"="", "Supported Models"="", "Instrument Options"="", "Flags"=0, "Help"="Returns the sample rate, that is the number of recorded waveform samples per second.\n\nAvailable Repeated Capabilities:\nNone\n\nRemote-control command(s):\nACQuire:SRATe?"}, {"Level"=2, "Class Only"=FALSE, "Identifier"="RSRTX_ATTR_AUTOSCALE", "Descriptive Name"="Autoscale", "Data Type"=4, "Command"="AUT", "Access"=1, "Range Table"="", "Read Callback"="", "Write Callback"="", "Supported Models"="", "Instrument Options"="", "Flags"=1, "Help"="Performs an autoset process: analyzes the enabled channel signals, and obtains appropriate horizontal, vertical, and trigger settings to display stable waveforms\n\nAvailable Repeated Capabilities:\nNone\n\nRemote-control command(s):\nAUToscale"}, {"Level"=2, "Class Only"=FALSE, "Identifier"="RSRTX_ATTR_HORZ_DIVISIONS", "Descriptive Name"="Horizontal Divisions", "Data Type"=1, "Command"="TIM:DIV?", "Access"=0, "Range Table"="", "Read Callback"="", "Write Callback"="", "Supported Models"="", "Instrument Options"="", "Flags"=0, "Help"="Queries the number of horizontal divisions on the screen. The number cannot be changed.\n\nAvailable Repeated Capabilities:\nNone\n\nRemote-control command(s):\nTIMebase:DIVisions?"}, {"Level"=2, "Class Only"=FALSE, "Identifier"="RSRTX_ATTR_HORZ_REFERENCE", "Descriptive Name"="Horizontal Reference", "Data Type"=1, "Command"="TIM:REF", "Access"=2, "Range Table"="rsrtx_rngHorzReference", "Read Callback"="", "Write Callback"="", "Supported Models"="", "Instrument Options"="", "Flags"=0, "Help"="Sets the reference point of the time scale in % of the display. The reference point defines which part of the waveform is shown. If the Trigger offset is zero, the trigger point matches the reference point.\n\nAvailable Repeated Capabilities:\nNone\n\nRemote-control command(s):\nTIMebase:REFerence"}, {"Level"=2, "Class Only"=FALSE, "Identifier"="RSRTX_ATTR_ROLL_MODE", "Descriptive Name"="Roll Mode", "Data Type"=3, "Command"="TIM:ROLL:ENAB", "Access"=2, "Range Table"="", "Read Callback"="", "Write Callback"="", "Supported Models"="", "Instrument Options"="", "Flags"=0, "Help"="Activates the automatic roll mode.\n\nAvailable Repeated Capabilities:\nNone\n\nRemote-control command(s):\nTIMebase:ROLL:ENABle"}, {"Level"=2, "Class Only"=FALSE, "Identifier"="RSRTX_ATTR_TIMESTAMPS_FILENAME", "Descriptive Name"="Timestamps Filename", "Data Type"=2, "Command"="EXP:ATAB:NAME", "Access"=2, "Range Table"="", "Read Callback"="", "Write Callback"="", "Supported Models"="", "Instrument Options"="", "Flags"=0, "Help"="Defines the path and filename of the acqisition timestamps file. The file format is CSV. If the file already exists, it will be overwritten.\n\nAvailable Repeated Capabilities:\nNone\n\nRemote-control command(s):\nEXPort:ATABle:NAME"}, {"Level"=2, "Class Only"=FALSE, "Identifier"="RSRTX_ATTR_TIMESTAMPS_SAVE", "Descriptive Name"="Timestamps Save", "Data Type"=4, "Command"="EXP:ATAB:SAVE", "Access"=1, "Range Table"="", "Read Callback"="", "Write Callback"="", "Supported Models"="", "Instrument Options"="", "Flags"=0, "Help"="Saves the acquisition timestamps table to the file that is defined by the EXPort:ATABle:NAME command.\n\nAvailable Repeated Capabilities:\nNone\n\nRemote-control command(s):\nEXPort:ATABle:SAVE"}, {"Level"=2, "Class Only"=TRUE, "Identifier"="", "Descriptive Name"="Channel", "Data Type"=0, "Command"="", "Access"=0, "Range Table"="", "Read Callback"="", "Write Callback"="", "Supported Models"="", "Instrument Options"="", "Flags"=0, "Help"="This class contains attributes that configure the channel acquisition subsystem."}, {"Level"=3, "Class Only"=FALSE, "Identifier"="RSRTX_ATTR_ACQUISITION_TYPE", "Descriptive Name"="Acquisition Type", "Data Type"=0, "Command"="CHAN{Channel}:TYPE", "Access"=2, "Range Table"="rsrtx_rngAcquisitionType", "Read Callback"="", "Write Callback"="", "Supported Models"="", "Instrument Options"="", "Flags"=0, "Help"="Selects the method to reduce the data stream of the ADC to a stream of waveform points with lower sample rate.\n\nAvailable Repeated Capabilities:\nChannel: CH0, CH1, CH2, CH3, CH4, CHExt\r\n\nRemote-control command(s):\nCHANnel<m>:TYPE"}, {"Level"=3, "Class Only"=FALSE, "Identifier"="RSRTX_ATTR_WAVEFORM_ACQUISITION_TYPE", "Descriptive Name"="Waveform Acquisition Type", "Data Type"=0, "Command"="CHAN{Channel}:ARIT", "Access"=2, "Range Table"="rsrtx_rngWaveformArithmetics", "Read Callback"="", "Write Callback"="", "Supported Models"="", "Instrument Options"="", "Flags"=0, "Help"="Selects the method to reduce the data stream of the ADC to a stream of waveform points with lower sample rate.\n\nAvailable Repeated Capabilities:\nChannel: CH0, CH1, CH2, CH3, CH4, CHExt\r\n\nRemote-control command(s):\nCHANnel<m>:ARIThmetics"}, {"Level"=3, "Class Only"=FALSE, "Identifier"="RSRTX_ATTR_HORZ_RECORD_LENGTH", "Descriptive Name"="Horizontal Record Length", "Data Type"=0, "Command"="CHAN{Channel}:DATA:POIN", "Access"=1, "Range Table"="rsrtx_rngWaveformSamplesRange", "Read Callback"="", "Write Callback"="", "Supported Models"="", "Instrument Options"="", "Flags"=0, "Help"="Selects a range of samples that will be returned\n\nAvailable Repeated Capabilities:\nChannel: CH0, CH1, CH2, CH3, CH4, CHExt\r\n\nRemote-control command(s):\nCHANnel<m>:DATA:POINts"}, {"Level"=3, "Class Only"=FALSE, "Identifier"="RSRTX_ATTR_GET_HORZ_RECORD_LENGTH", "Descriptive Name"="Get Horizontal Record Length", "Data Type"=0, "Command"="CHAN{Channel}:DATA:POIN?", "Access"=0, "Range Table"="", "Read Callback"="", "Write Callback"="", "Supported Models"="", "Instrument Options"="", "Flags"=0, "Help"="Returns the horizontal record length.\n\nAvailable Repeated Capabilities:\nChannel: CH0, CH1, CH2, CH3, CH4, CHExt\r\n\nRemote-control command(s):\nCHANnel<m>:DATA:POINts?"}, {"Level"=1, "Class Only"=TRUE, "Identifier"="", "Descriptive Name"="Probe", "Data Type"=0, "Command"="", "Access"=0, "Range Table"="", "Read Callback"="", "Write Callback"="", "Supported Models"="", "Instrument Options"="", "Flags"=0, "Help"="This class contains attributes that configure the probe subsystem."}, {"Level"=2, "Class Only"=FALSE, "Identifier"="RSRTX_ATTR_PROBE_TYPE", "Descriptive Name"="Probe Type", "Data Type"=2, "Command"="PROB{Channel}:SET:TYPE?", "Access"=0, "Range Table"="", "Read Callback"="", "Write Callback"="", "Supported Models"="RTM|RTA", "Instrument Options"="", "Flags"=0, "Help"="Queries the type of the probe.\n\nAvailable Repeated Capabilities:\nChannel: CH0, CH1, CH2, CH3, CH4, CHExt\r\n\nRemote-control command(s):\nPROBe<m>:SETup:TYPE?"}, {"Level"=2, "Class Only"=FALSE, "Identifier"="RSRTX_ATTR_PROBE_NAME", "Descriptive Name"="Probe Name", "Data Type"=2, "Command"="PROB{Channel}:SET:NAME?", "Access"=0, "Range Table"="", "Read Callback"="", "Write Callback"="", "Supported Models"="", "Instrument Options"="", "Flags"=0, "Help"="Queries the name of the probe.\n\nAvailable Repeated Capabilities:\nChannel: CH0, CH1, CH2, CH3, CH4, CHExt\r\n\nRemote-control command(s):\nPROBe<m>:SETup:NAME?"}, {"Level"=2, "Class Only"=FALSE, "Identifier"="RSRTX_ATTR_PROBE_INPUT_IMPEDANCE", "Descriptive Name"="Probe Input Impedance", "Data Type"=0, "Command"="PROB{Channel}:SET:IMP?", "Access"=0, "Range Table"="rsrtx_rngProbeInputImpedance", "Read Callback"="", "Write Callback"="", "Supported Models"="RTM|RTA", "Instrument Options"="", "Flags"=0, "Help"="Queries the termination of the probe.\n\nAvailable Repeated Capabilities:\nChannel: CH0, CH1, CH2, CH3, CH4, CHExt\r\n\nRemote-control command(s):\nPROBe<m>:SETup:IMPedance?"}, {"Level"=2, "Class Only"=FALSE, "Identifier"="RSRTX_ATTR_PROBE_INPUT_CAPACITANCE", "Descriptive Name"="Probe Input Capacitance", "Data Type"=1, "Command"="PROB{Channel}:SET:CAP?", "Access"=0, "Range Table"="", "Read Callback"="", "Write Callback"="", "Supported Models"="RTM|RTA", "Instrument 
